vi "Get Temp Class Name.vi"(11 "Mock Class Generator Test in":refnum<class "Pure Mock Class Generator Test.lvclass">) -> (3 "Test Class Path":path)   [LabVIEW 2020, in "Pure Mock Class Generator Test.lvclass"]
uses:
  Pure Mock Class Generator Test.lvclass
  Pure Mock Class Generator Test.lvclass/Pure Mock Class Generator Test.ctl
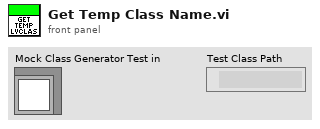
[diagram p1: front panel]
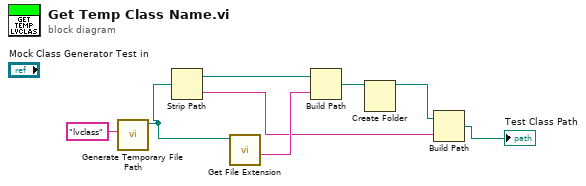
[diagram p0: block diagram]
diagram:
  n1 = call <vilib>:"Generate Temporary File Path.vi"("Temporary File Extension (tmp)"="lvclass") -> ("Unique Temporary File Path"=w7:path)  [unwired: 9 in, 1 out]
  n2 = Strip Path(path=w7) -> (stripped path=w6:path, name=w3:string)
  n3 = call <vilib>:"Get File Extension.vi"("file"=w7) -> ("filename without extension"=w5:string)  [unwired: 6 in, 4 out]
  n4 = Build Path(base path=w6, name or relative path=w5) -> (appended path=w4:path)
  n5 = Create Folder(path (use dialog)=w4) -> (created path=w1:path)  [unwired: 2 in, 2 out]
  n6 = Build Path(base path=w1, name or relative path=w3) -> (appended path=→"Test Class Path":path)
